vi "tenma_voltage.vi"(7 "override":bool, 8 "error in (no error)":errorcluster, 10 "voltage (V)":dbl format="%#_16g", 11 "VISA IN":refnum<visa-resource-name>) -> (0 "error out":errorcluster, 2 "value out":dbl=0.000301 format="%#_16p")   [LabVIEW 2017]
uses:
  hardware/tenma/tenma.lvlib
panel:
  in  "lower limit":dbl format="%#_13g"
  in  "upper limit":dbl=5.0 format="%#_13g"
  in  "VISA (default)":refnum<visa-resource-name>="Tenma"
  # "Tenma 72-2540\nNb.  0 V = output OFF."
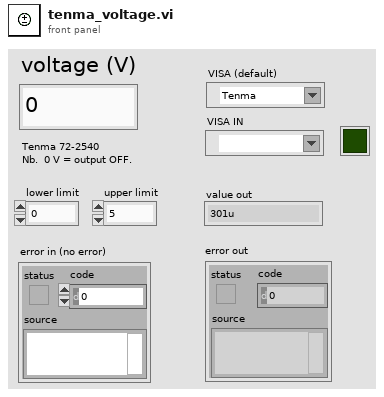
[diagram p1: front panel]
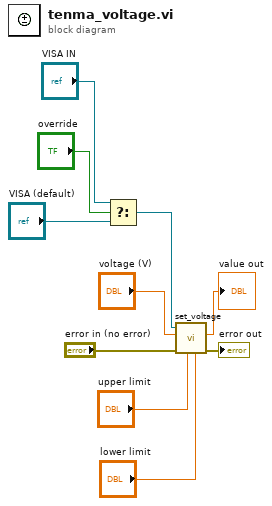
[diagram p0: block diagram]
diagram:
  n1 = Select(t="VISA IN", s="override", f="VISA (default)") -> (s? t:f=w5:refnum<visa-resource-name>)
  n2 = call "set_voltage.vi"("lower limit"="lower limit", "upper limit"="upper limit", "error in (no error)"="error in (no error)", "value"="voltage (V)", "VISA resource name"=w5) -> ("error out"=→"error out":errorcluster, "value_out"=→"value out":dbl)  [unwired: 4 in, 1 out]
